vi "Read Measurement (Carrier Power - Frequency).vi"(8 "error in (no error)":errorcluster, 9 "Maximum Time (25000 ms)":i32=25000, 11 "VISA resource name":refnum<visa-resource-name>) -> (0 "error out":errorcluster, 1 "Carrier Frequency (Hz)":dbl, 2 "Carrier Power (dBm)":dbl, 3 "VISA resource name out":refnum<visa-resource-name>)   [LabVIEW 2014, in "Agilent ESA PSA Series.lvlib"]
doc: "Stops the present measurement and sets up the instrument for a log plot or spot frequency, carrier power and carrier frequency measurement.\n\nAfter the data are valid, the result is returned for the specified measurement. These are the settings and units that conform to the measurement specific standard.\n\n- Stops the current measurement and does not reset the measurement to the factory defaults. \n\n- Initiates the measurement and puts valid data into the output buffer. If a measurement other than the current one is specified, the instrument will switch to that measurement before it initiates the measurement and returns results.\n\n- Waits until the measurement is complete before returning results.\n\n<B>Note:</B> \n\nThis VI is valid for both Spot Frequency and Log Plot functionalities of the Phase Noise personality."
uses:
  Agilent ESA PSA Series.lvlib
  Fetch Measurement (Carrier Power - Frequency).vi
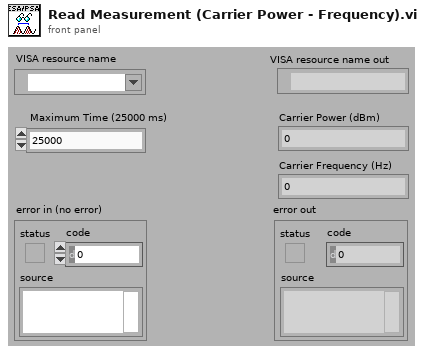
[diagram p1: front panel]
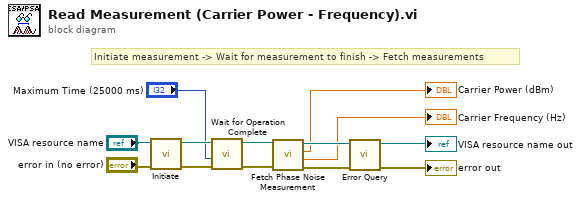
[diagram p0: block diagram]
diagram:
  # "Initiate measurement -> Wait for measurement to finish -> Fetch measurements"
  n1 = call "Initiate.vi"("error in (no error)"="error in (no error)", "VISA resource name"="VISA resource name") -> ("error out"=w2:errorcluster, "VISA resource name out"=w3:refnum<visa-resource-name>)  [unwired: 8 in]
  n2 = call "Wait for Operation Complete.vi"("error in (no error)"=w2, "Maximum Time (10000ms)"="Maximum Time (25000 ms)", "VISA resource name"=w3) -> ("error out"=w10:errorcluster, "VISA resource name out"=w11:refnum<visa-resource-name>)  [unwired: 7 in]
  n3 = call-poly "Fetch Phase Noise Measurement.vi"("error in (no error)"=w10, "VISA resource name"=w11) -> ("error out"=w8:errorcluster, "Carrier Frequency (Hz)"=→"Carrier Frequency (Hz)":dbl, "Carrier Power (dBm)"=→"Carrier Power (dBm)":dbl, "VISA resource name out"=w9:refnum<visa-resource-name>)  [unwired: 6 in]
  n4 = call "Error Query.vi"("error in (no error)"=w8, "VISA resource name"=w9) -> ("error out"=→"error out":errorcluster, "VISA resource name out"=→"VISA resource name out":refnum<visa-resource-name>)  [unwired: 6 in, 2 out]
